vi "ProdaNG.ProductComponent.Get.vi"(8 "error in (no error)":errorcluster, 9 "serialNumber":string, 10 "wabcoNumber":string, 11 "dbHandle":i32) -> (0 "error out":errorcluster, 2 "ProdComponents":T1[](array[typedef]), 3 "dbHandle out":i32)   [LabVIEW 2016]
doc: "This function returns a product structure for a product, which is identified by a part and a serial number.\nImportant information: The field 'individual' was taken over from the field 'allgemein' of the legacy data directly. Because of this most products have the value 0 further on and only a few the value 1. \nParameter:\nhandle is an Integer, which is returned by the function Login() at the creation of a new connection.\nwabcoPartId is the Id of the part.\nserialNumber is the serial number of the product for the part above.\nproduct is a pointer on a product structure, which is filled if the returncode is 0. The structure must be defined in the calling program.\n\nReturncodes:\n0 No error\n< 0 ORACLE Error code\n6 (ERROR_INVALID_HANDLE) in case of an invalid handle\n1403 Record does not exist"
uses:
  Controls/ProdaNG.ProductComponent.ctl
  Controls/ProdaNG.ProductionLineSize.ctl
  <vilib>/Utility/importsl/GetValueByPointer/datatype.ctl
  <vilib>/Utility/importsl/GetValueByPointer/GetValueByPointer.xnode
  prodllNG.dll
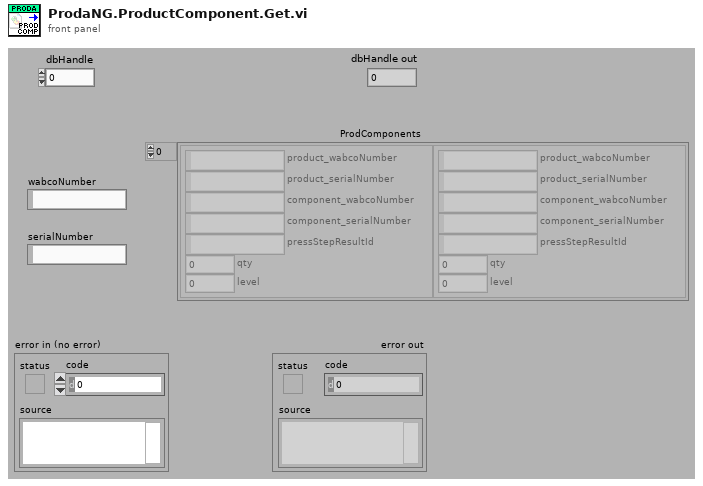
[diagram p1: front panel]
types:
  T1 = typedef "ProdaNG.ProductComponent.ctl" = cluster{"product_wabcoNumber":string, "product_serialNumber":string, "component_wabcoNumber":string, "component_serialNumber":string, "pressStepResultId":string, "qty":i32, "level":i32}
  T2 = typedef "ProdaNG.ProductionLineSize.ctl" = cluster{"product_wabcoNumber":i32, "product_serialNumber":i32, "component_wabcoNumber":i32, "component_serialNumber":i32, "pressStepResultId":i32, "qty":i32, "level":i32}
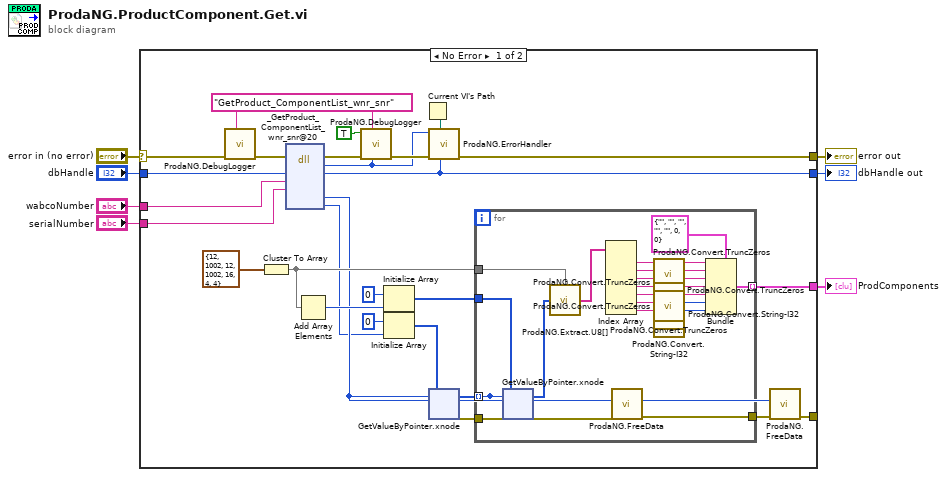
[diagram p0: block diagram]
diagram:
  n1 = case shown="No Error" "error in (no error)" {
    selector: "error in (no error)" -> [w32 w90]
    tunnel: [w33 w90] -> w6
    tunnel: "dbHandle" -> [w26 w89]
    tunnel: [w27 w89] -> w4
    tunnel: "wabcoNumber" -> [w28 _]
    tunnel: "serialNumber" -> [w29 _]
    tunnel: [w10 _] -> w1
    tunnel: [w9 _] -> _
    frame No Error {
      w22 = "GetProduct_ComponentList_wnr_snr" ("cmd")
      n2 = call "ProdaNG.DebugLogger.vi"("cmd"=w22, "error in (no error)"=w32) -> ("error out"=w25:errorcluster)  [unwired: 9 in]
      n3 = Cluster To Array(cluster=T2 {"product_wabcoNumber"=12, "product_serialNumber"=1002, "component_wabcoNumber"=12, "component_serialNumber"=1002, "pressStepResultId"=16, "qty"=4, "level"=4} ("ProductComponentSize")) -> (array=w14:i32[])
      n4 = dll-call lib="D:/Maszup/WABCO/SVN/LineTraceSystem/SOFTWARE/sources/Database/ProdaNG/prodllNG.dll" fn="_GetProduct_ComponentList_wnr_snr@20" ("ProDll wrapper.dll:wrapper_GetWabcoParts_init")(error in=w25, "dbHandle"=w26, "wabcoNumber"=w28, "serialNumber"=w29) -> (error out=w24:errorcluster, "return type"=w30:i32, "dbHandle"=w27:i32, "product_component_wnr_snr"=w11:i32, "countPtr"=w8:u32)  [unwired: 6 in, 1 out]
      n5 = Add Array Elements(numeric array=w14) -> (sum=w15:i32)
      n6 = call "ProdaNG.DebugLogger.vi"("return type"=w30, "cmd"=w22, "error in (no error)"=w24, "done? (F)"=TRUE) -> ("error out"=w31:errorcluster)  [unwired: 7 in]
      n7 = Initialize Array(u8 0 ("element"), w15) -> (w16:u8[])
      n8 = Initialize Array(u32 0 ("element"), w8) -> (w21:u32[])
      n9 = Current VI's Path() -> (path=w34:path)
      n10 = call "ProdaNG.ErrorHandler.vi"("dbHandleIn"=w27, "Path"=w34, "error in"=w31, "output_parameter"=w30) -> ("error out"=w33:errorcluster)  [unwired: 7 in]
      n11 = xnode "GetValueByPointer.xnode"("Pointer"=w11, "InputType"=w21) -> ("Output"=w18:u32[], "ErrorOut"=w19:errorcluster)  [unwired: 2 in]
      n12 = for {
        tunnel: w19 -> [w58]
        tunnel: w18 -> [w38] mode=indexing
        tunnel: w16 -> [w57]
        tunnel: w14 -> [w41]
        tunnel: [w40] -> w10 mode=indexing
        tunnel: [w37] -> w13
        n13 = xnode "GetValueByPointer.xnode"("Pointer"=w38, "InputType"=w57, "ErrorIn"=w58) -> ("Output"=w43:u8[], "ErrorOut"=w39:errorcluster)  [unwired: 1 in]
        n14 = call "ProdaNG.Extract.U8[].vi"("unsigned byte array"=w43, "Sizes"=w41) -> ("Elements"=w42:string[])
        n15 = Index Array(array=w42) -> (element #1=w45:string, element #2=w44:string, element #3=w55:string, element #4=w52:string, element #5=w49:string, element #6=w51:string, element #7=w35:string)  [unwired: 7 in]
        n16 = call "ProdaNG.FreeData.vi"("error in (no error)"=w39, "Pointers"=w38) -> ("error out"=w37:errorcluster)  [unwired: 9 in]
        n17 = call "ProdaNG.Convert.TruncZeros.vi"("string with \\0s"=w45) -> ("LV string"=w47:string)  [unwired: 10 in]
        n18 = call "ProdaNG.Convert.TruncZeros.vi"("string with \\0s"=w44) -> ("LV string"=w46:string)  [unwired: 10 in]
        n19 = call "ProdaNG.Convert.TruncZeros.vi"("string with \\0s"=w55) -> ("LV string"=w54:string)  [unwired: 10 in]
        n20 = call "ProdaNG.Convert.TruncZeros.vi"("string with \\0s"=w52) -> ("LV string"=w53:string)  [unwired: 10 in]
        n21 = call "ProdaNG.Convert.TruncZeros.vi"("string with \\0s"=w49) -> ("LV string"=w48:string)  [unwired: 10 in]
        n22 = call "ProdaNG.Convert.String-I32.vi"("unsigned byte string"=w51) -> ("32bit integer"=w50:i32)  [unwired: 10 in]
        n23 = call "ProdaNG.Convert.String-I32.vi"("unsigned byte string"=w35) -> ("32bit integer"=w36:i32)  [unwired: 10 in]
        n24 = Bundle(cluster=T1 {"product_wabcoNumber"="", "product_serialNumber"="", "component_wabcoNumber"="", "component_serialNumber"="", "pressStepResultId"="", "qty"=0, "level"=0} ("Product_Component_wnr_str"), "product_wabcoNumber"=w47, "product_serialNumber"=w46, "component_wabcoNumber"=w54, "component_serialNumber"=w53, "pressStepResultId"=w48, "qty"=w50, "level"=w36) -> (w40:T1)
      }
      n25 = call "ProdaNG.FreeData.vi"("error in (no error)"=w13, "Pointers"=w11) -> ("error out"=w9:errorcluster)  [unwired: 9 in]
    }
    frame Error {
    }
  }
  "error out" <- w6
  "dbHandle out" <- w4
  "ProdComponents" <- w1
